vi "미니 상태 머신 알고리즘 실습.vi"() -> ()   [LabVIEW 2020]
panel:
  in  "s":bool
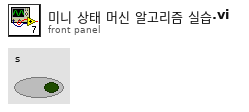
[diagram p1: front panel]
types:
  T1 = typedef "상태 컨트롤.ctl" = enum16{"시작", "대기", "종료"}
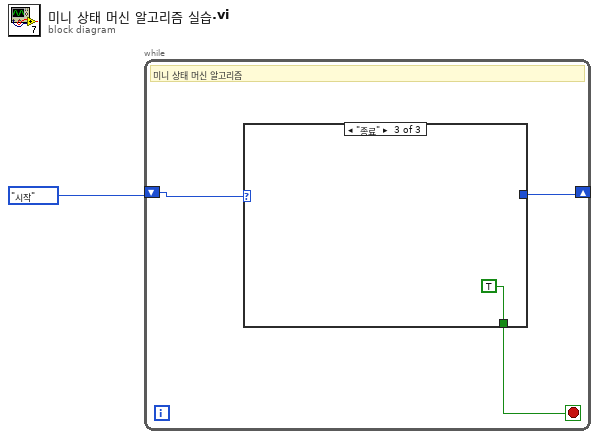
[diagram p0: block diagram]
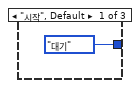
[diagram p2: hidden frame]
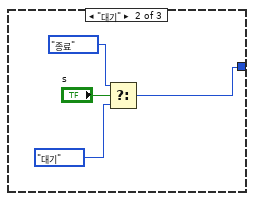
[diagram p3: hidden frame]
diagram:
  n1 = while {
    shift-right: [w3] -> _
    shift-left: 상태_컨트롤."시작" -> [w4]
    stop <- w2 stop-if-true
    # "미니 상태 머신 알고리즘"
    n2 = case shown="\"종료\"" w4 {
      tunnel: [상태_컨트롤."대기" w6 _] -> w3
      tunnel: [_ _ TRUE] -> w2
      frame "시작", Default {
      }
      frame "대기" {
        n3 = Select(t=상태_컨트롤."종료", s="s", f=상태_컨트롤."대기") -> (s? t:f=w6:T1)
      }
      frame "종료" {
      }
    }
  }
